vi "Pre Launch Init.vi"(11 "Nested in":refnum<class "RefNums and UICtrl.lvclass">) -> (0 "error out":errorcluster, 3 "Nested out":refnum<class "RefNums and UICtrl.lvclass">)   [LabVIEW 2020, in "RefNums and UICtrl.lvclass"]
doc: "(<B>Filename</B>: Actor Framework.lvlib:Actor.lvclass:Pre Launch Init.vi)\n\nDefines behavior that occurs after the Launch Nested Actor method is invoked but before the actor's Actor Core method begins running.\n\nBy default, this method does nothing. A descendant class may override it to define behavior."
uses:
  RefNums and UICtrl.lvclass
  RefNums and UICtrl.lvclass/RefNums and UICtrl.ctl
  <vilib>/MGI/Monitored Actor/Monitored Actor/Monitored Actor/Monitored Actor.lvclass
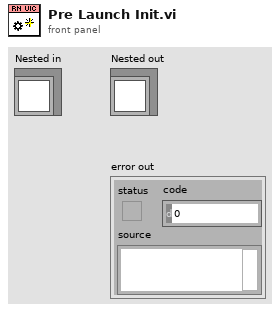
[diagram p1: front panel]
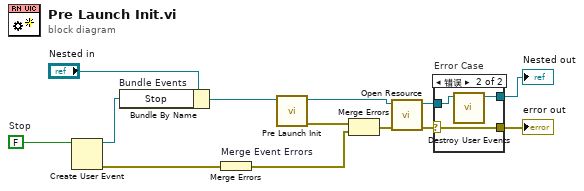
[diagram p0: block diagram]
diagram:
  w12 = FALSE  # Stop
  n1 = Create User Event(user event datatype=w12) -> (user event=w9:refnum<user-event>, error out=w11:errorcluster)  [unwired: 1 in]
  n2 = Bundle By Name "Bundle Events"(cluster="Nested in", "Stop"=w9) -> (w7:refnum<class "RefNums and UICtrl.lvclass">)
  n3 = Merge Errors "Merge Event Errors"(w11) -> (w4:errorcluster)
  n4 = call-parent "Pre Launch Init.vi"("Monitored Actor in"=w7) -> ("error out"=w6:errorcluster, "Monitored Actor out"=w2:refnum<class "RefNums and UICtrl.lvclass">)  [unwired: 9 in]
  n5 = Merge Errors ("合并错误")(w6, w4) -> (w5:errorcluster)
  n6 = call "Open Resource.vi"("error in (no error)"=w5, "Nested in"=w2) -> ("error out"=w3:errorcluster, "Nested out"=w1:refnum<class "RefNums and UICtrl.lvclass">)  [unwired: 8 in]
  n7 = case "Error Case" shown="错误" w3 {
    selector: w3 -> [w14 w18]
    tunnel: w1 -> [w15 w17]
    tunnel: [w15 w16] -> w10
    tunnel: [w14 w18] -> w8
    frame No Error {
    }
    frame Error {
      n8 = call "Destroy User Events.vi"("Nested in"=w17) -> ("Nested out"=w16:refnum<class "RefNums and UICtrl.lvclass">)  [unwired: 10 in]
    }
  }
  "error out" <- w8
  "Nested out" <- w10
